vi "Query Calibration Date.vi"(0 "VISA resource name":refnum<visa-resource-name>, 11 "error in (no error)":errorcluster) -> (4 "VISA resource name out":refnum<visa-resource-name>, 6 "Time Stamp":timestamp format="%<%X\n%x>T", 15 "error out":errorcluster)   [LabVIEW 2020, in "NH Research Regenerative Test Series.lvlib"]
doc: "Returns the last date the calibration factors were saved to flash."
uses:
  Drivers-Essentials/NH Research Regenerative Test Series.lvlib
  <vilib>/Utility/miscctls.llb/LVDateTimeRec.ctl
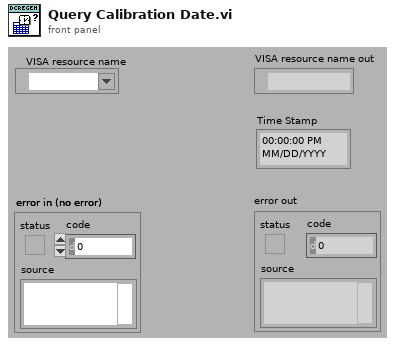
[diagram p1: front panel]
types:
  T1 = typedef "LVDateTimeRec.ctl" = cluster{"fractional second":dbl, "second":i32, "minute":i32, "hour":i32, "day of month":i32, "month":i32, "year":i32, "day of week":i32, "day of year":i32, "DST":i32}
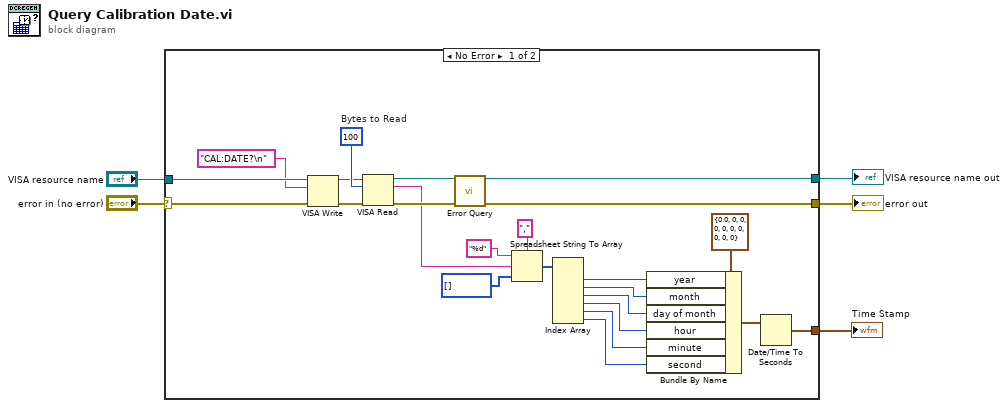
[diagram p0: block diagram]
diagram:
  n1 = case shown="No Error" "error in (no error)" {
    selector: "error in (no error)" -> [w22 w31]
    tunnel: [w17 w31] -> w4
    tunnel: [w25 w30] -> w2
    tunnel: "VISA resource name" -> [w26 w30]
    tunnel: [w6 _] -> w1
    frame No Error {
      w29 = u32 100  # Bytes to Read
      n2 = VISA Write(VISA resource name=w26, write buffer="CAL:DATE?\n" ("Command"), error in (no error)=w22) -> (VISA resource name out=w27:refnum<visa-resource-name>, error out=w28:errorcluster)  [unwired: 1 out]
      n3 = VISA Read(VISA resource name=w27, byte count=w29, error in (no error)=w28) -> (VISA resource name out=w24:refnum<visa-resource-name>, read buffer=w16:string, error out=w23:errorcluster)  [unwired: 1 out]
      n4 = call "Error Query.vi"("VISA resource name"=w24, "error in (no error)"=w23) -> ("VISA resource name out"=w25:refnum<visa-resource-name>, "error out"=w17:errorcluster)  [unwired: 10 in, 2 out]
      n5 = Spreadsheet String To Array(delimiter (Tab)=",", format string="%d", spreadsheet string=w16, array type (2D Dbl)=i32[] []) -> (array=w14:i32[])
      n6 = Index Array(array=w14) -> (element #1=w13:i32, element #2=w12:i32, element #3=w11:i32, element #4=w10:i32, element #5=w9:i32, element #6=w8:i32)  [unwired: 6 in]
      n7 = Bundle By Name(cluster=T1 {"fractional second"=0.0, "second"=0, "minute"=0, "hour"=0, "day of month"=0, "month"=0, "year"=0, "day of week"=0, "day of year"=0, "DST"=0} ("date time rec"), "year"=w13, "month"=w12, "day of month"=w11, "hour"=w10, "minute"=w9, "second"=w8) -> (w7:T1)
      n8 = Date/Time To Seconds(2:w7) -> (0:w6:timestamp)  [unwired: 1 in]
    }
    frame Error {
    }
  }
  "error out" <- w4
  "VISA resource name out" <- w2
  "Time Stamp" <- w1
